vi "to string.vi"(8 "error in":errorcluster, 11 "configuration in":refnum<class "Bus Configuration.lvclass">) -> (0 "error out":errorcluster, 1 "data":string, 2 "version":string, 3 "configuration out":refnum<class "Bus Configuration.lvclass">)   [LabVIEW 2014, in "Bus Configuration.lvclass"]
doc: "Provides an interface for saving a module configuration to a file or other serialized data source. It is recommended that all children of this class store data in two sets--data required for its own initialization, and any data required for parent initialization--and that each implementation uses the <b>Call Parent Method</b> primitive to serialize parent information."
uses:
  Bus Configuration.lvclass
  Bus Configuration.lvclass/Bus Configuration.ctl
  <vilib>/NI/Configuration Framework/serializable configuration/NISE_CEF_serializable configuration.lvclass
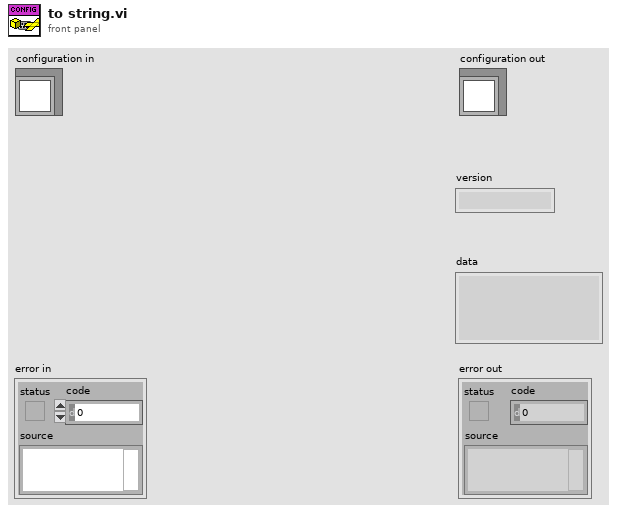
[diagram p1: front panel]
types:
  T1 = typedef "Bus Configuration.lvclass/SPI Configuration.ctl" = cluster{"SCLK":string, "MOSI":string, "MISO":string}
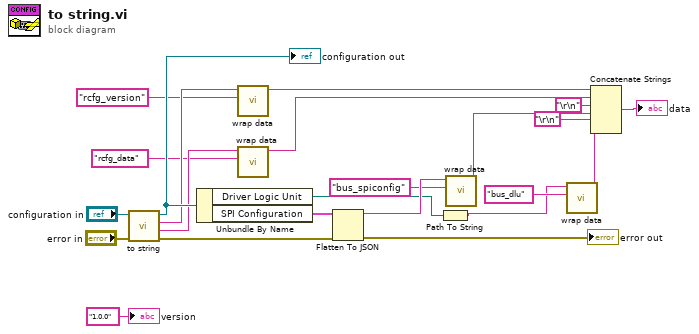
[diagram p0: block diagram]
diagram:
  n1 = call-parent "to string.vi"("error in"="error in", "configuration in"="configuration in") -> ("error out"=w19:errorcluster, "data"=w15:string, "version"=w16:string, "configuration out"=w21:refnum<class "Bus Configuration.lvclass">)  [unwired: 6 in]
  "configuration out" <- w21
  n2 = Unbundle By Name(w21) -> ("Driver Logic Unit"=w3:path, "SPI Configuration"=w20:T1)
  n3 = call <vilib>:"wrap data.vi"("identifier"="rcfg_version", "data to wrap"=w16) -> ("wrapped data"=w11:string)  [unwired: 9 in]
  n4 = call <vilib>:"wrap data.vi"("identifier"="rcfg_data", "data to wrap"=w15) -> ("wrapped data"=w10:string)  [unwired: 9 in]
  n5 = Flatten To JSON(anything=w20, error in (no error)=w19) -> (JSON string=w18:string, 11:→"error out":errorcluster)  [unwired: 1 in]
  n6 = Path To String(path=w3) -> (string=w2:string)
  n7 = call <vilib>:"wrap data.vi"("identifier"="bus_spiconfig", "data to wrap"=w18) -> ("wrapped data"=w8:string)  [unwired: 9 in]
  n8 = call <vilib>:"wrap data.vi"("identifier"="bus_dlu", "data to wrap"=w2) -> ("wrapped data"=w4:string)  [unwired: 9 in]
  n9 = Concatenate Strings(w11, w10, "\r\n", w8, "\r\n", w4) -> (→"data":string)
  "version" <- "1.0.0" ("version")
